vi "Dispenser Control.vi"() -> ()   [LabVIEW 2016]
uses:
  GitHub/UCSB-Gantry/V5/Drivers/EFD Ultimus V/EFD Ultimus V.lvlib
panel:
  in  "Go":bool
  in  "Dispense for 5 sec":bool
  in  "stop":bool
  in  "Dispense\nOn/Off":bool
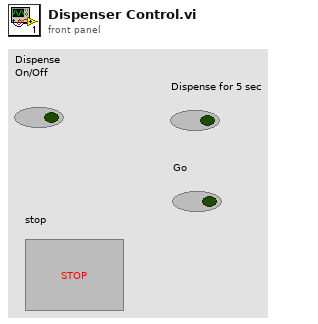
[diagram p1: front panel]
types:
  T1 = cluster{"Baud Rate ":u32, "Parity ":u16, "Data Bits ":u16, "Stop Bits":u16}
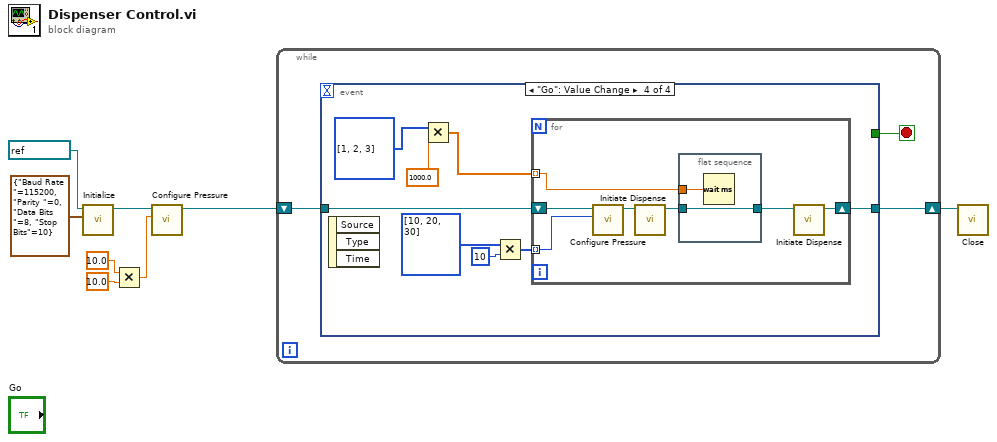
[diagram p0: block diagram]
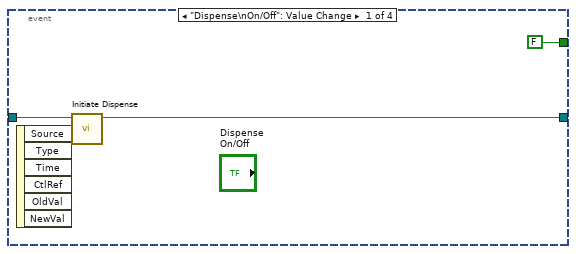
[diagram p2: hidden frame]
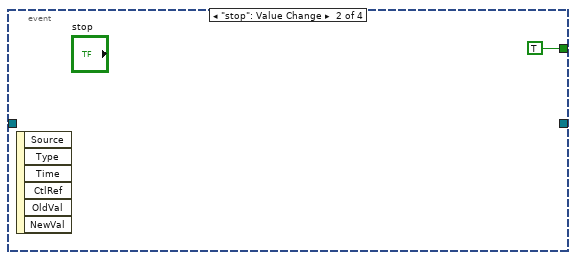
[diagram p3: hidden frame]
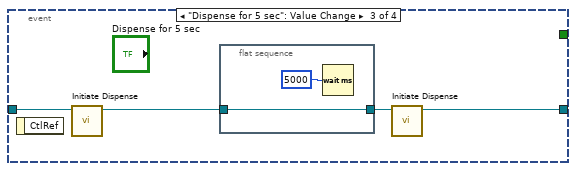
[diagram p4: hidden frame]
diagram:
  n1 = call "Initialize.vi"("Serial Configuration"=T1 {"Baud Rate "=115200, "Parity "=0, "Data Bits "=8, "Stop Bits"=10}, "VISA resource name"=refnum<visa-resource-name> "COM1") -> ("VISA resource name out"=w6:refnum<visa-resource-name>)  [unwired: 8 in, 1 out]
  n2 = Multiply(x=10.0, y=10.0) -> (x*y=w2:dbl)
  n3 = call "Configure Pressure.vi"("Pressure Setting (0000)"=w2, "VISA resource name"=w6) -> ("VISA resource name out"=w5:refnum<visa-resource-name>)  [unwired: 8 in, 1 out]
  n4 = while {
    shift-right: [w10] -> w1
    shift-left: w5 -> [w11]
    stop <- w9 stop-if-true
    n5 = event shown="[3] \"Go\": Value Change" {
      selector: _ -> [_ _ _ _]
      dyn-events: _ -> [_ _ _ _]
      timeout: _ -> [_ _ _ _]
      tunnel: w11 -> [w14 _ w19 w29]
      tunnel: [w13 _ w16 w28] -> w10
      tunnel: [FALSE TRUE _ _] -> w9
      event "Dispense\nOn/Off": Value Change {
        n6 = event-data() -> ()  [unwired: 1 in, 6 out]
        n7 = call "Initiate Dispense.vi"("VISA resource name"=w14) -> ("VISA resource name out"=w13:refnum<visa-resource-name>)  [unwired: 9 in, 1 out]
      }
      event "stop": Value Change {
        n8 = event-data() -> ()  [unwired: 1 in, 6 out]
      }
      event "Dispense for 5 sec": Value Change {
        n9 = event-data() -> ()  [unwired: 1 in, 1 out]
        n10 = call "Initiate Dispense.vi"("VISA resource name"=w19) -> ("VISA resource name out"=w18:refnum<visa-resource-name>)  [unwired: 9 in, 1 out]
        n11 = flat-sequence {
          tunnel: w18 -> [w20]
          tunnel: [w20] -> w17
          frame #0 {
            n12 = Wait (ms)(milliseconds to wait=u32 5000) -> ()  [unwired: 1 out]
          }
        }
        n13 = call "Initiate Dispense.vi"("VISA resource name"=w17) -> ("VISA resource name out"=w16:refnum<visa-resource-name>)  [unwired: 9 in, 1 out]
      }
      event "Go": Value Change {
        n14 = event-data() -> ()  [unwired: 1 in, 3 out]
        n15 = Multiply(x=i32[] [1, 2, 3], y=1000.0) -> (x*y=w22:dbl[])
        n16 = Multiply(x=i32[] [10, 20, 30], y=10) -> (x*y=w25:i32[])
        n17 = for {
          shift-right: [w33] -> w28
          shift-left: w29 -> [w31]
          tunnel: w22 -> [w36] mode=indexing
          tunnel: w25 -> [w32] mode=indexing
          n18 = call "Configure Pressure.vi"("Pressure Setting (0000)"=w32, "VISA resource name"=w31) -> ("VISA resource name out"=w30:refnum<visa-resource-name>)  [unwired: 8 in, 1 out]
          n19 = call "Initiate Dispense.vi"("VISA resource name"=w30) -> ("VISA resource name out"=w35:refnum<visa-resource-name>)  [unwired: 9 in, 1 out]
          n20 = flat-sequence {
            tunnel: w36 -> [w38]
            tunnel: w35 -> [w37]
            tunnel: [w37] -> w34
            frame #0 {
              n21 = Wait (ms)(milliseconds to wait=w38) -> ()  [unwired: 1 out]
            }
          }
          n22 = call "Initiate Dispense.vi"("VISA resource name"=w34) -> ("VISA resource name out"=w33:refnum<visa-resource-name>)  [unwired: 9 in, 1 out]
        }
      }
    }
  }
  n23 = call "Close.vi"("VISA resource name"=w1) -> ()  [unwired: 10 in, 1 out]
